vi "T6_E4980A_Correction.vi"(4 "Cable Length (0: 0 m)":u16(ring)=2 items=["0 m"=0, "1 m"=1, "2 m"=2, "4 m"=4], 5 "LCR Correction String":string="CORR:LENG 1;METH MULT;OPEN:STAT ON;:CORR:SHOR:STAT OFF;:CORR:LOAD:STAT OFF;:CORR:SPOT1:STAT ON;FREQ 2E6", 6 "Calib waitTime (ms)":u32=1000, 7 "LCR Setup String":string="FUNC:IMP:TYPE CPQ;RANG:AUTO ON;:FREQ 8E5;VOLT 1;TRIG:SOUR INT;:AMPL:ALC OFF;:APER SHORT,4", 8 "error in":errorcluster, 9 "Relay Definition for Path":string[](array[string])=["C10,C26,C42,C58", "O10,O26,C30,O42,O58,C63", "O10,O26,C30,O42,O58,C63", "O10,O26,C30,O42,O58,C63", "C14,C28,O30,C40,C47,C52,C60,O63", "O14,O28,C31,C40,O47,C52,C54,O60", "C15,C31,C40,C52,C54,C56", "O15,O31,C28,C40,O54,O56,C52,C60", "C28,C40,C52,C60", "C28,C40,C52,C60", "C11,O28,C30,O40,C43,O52,O60,C63", "O11,C26,O30,O43,C58,O63", "C9,O26,C41,O58", "O9,O26,C27,C30,O41,C59,C63", "C13,O27,O30,C40,C46,C52,O59,O63", "C13,C40,C46,C52", "C13,C40,C46,C52", "O13,C29,C31,C40,C52,C54,C61,O46", "C24,C29,C31,C40,C52,C54,C57,C61", "O24,O29,O31,C40,O54,C52,O57,O61", "C12,C27,C30,O40,C44,C59,O52,C63", "C12,C27,C30,O40,C44,C59,O52,C63", "C12,C27,C30,O40,C44,C59,O52,C63", "O9,O26,O10,O36,O11,O27,O12,O40,O14,O31,O13,O28,O15,O29,O24,O41,O58,O42,O60,O63,O43,O59,O44,O52,O46,O60,O47,O54,O56,O61,O57", "C38"], 10 "LCR Meter In":refnum<visa-resource-name>="GPIB0::17::INSTR", 11 "Relay In":refnum<k15>="PXI1Slot2" caption="resource name") -> (0 "error out (no error)":errorcluster, 2 "LCR Out":refnum<visa-resource-name>, 3 "Relay Out":refnum<k15>)   [LabVIEW 2017]
uses:
  <instrlib>/Agilent E4980/Agilent E4980.lvlib
panel:
  in  "T6_Relay Definition for Path":string[](array[string])=["C10,C26,C42,C58", "O10,O26,C30,O42,O58,C63", "C11,O28,C30,O40,C43,O52,O60,C63", "O11,C26,O30,O43,C58,O63", "C38", "O14,O28,C31,C40,O47,C52,C54,O60", "C15,C31,C40,C52,C54,C56", "O15,O31,C28,C40,O54,O56,C52,C60", "C28,C40,C52,C60", "C28,C40,C52,C60", "C11,O28,C30,O40,C43,O52,O60,C63", "O11,C26,O30,O43,C58,O63", "C9,O26,C41,O58", "O9,O26,C27,C30,O41,C59,C63", "C13,O27,O30,C40,C46,C52,O59,O63", "C13,C40,C46,C52", "C13,C40,C46,C52", "O13,C29,C31,C40,C52,C54,C61,O46", "C24,C29,C31,C40,C52,C54,C57,C61", "O24,O29,O31,C40,O54,C52,O57,O61", "C12,C27,C30,O40,C44,C59,O52,C63", "C12,C27,C30,O40,C44,C59,O52,C63", "C12,C27,C30,O40,C44,C59,O52,C63", "O9,O26,O10,O36,O11,O27,O12,O40,O14,O31,O13,O28,O15,O29,O24,O41,O58,O42,O60,O63,O43,O59,O44,O52,O46,O60,O47,O54,O56,O61,O57", "C38"]
  # "Spot 1 --> TMN1.5\nSpot 2 --> VMD"
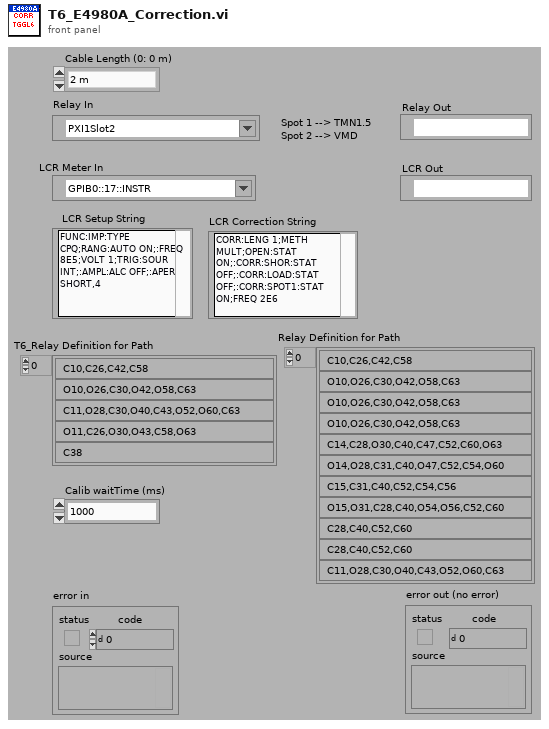
[diagram p1: front panel]
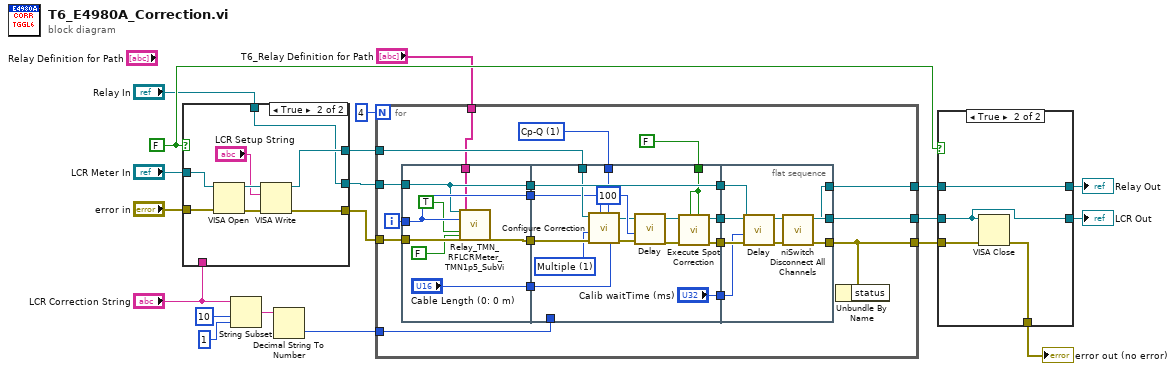
[diagram p0: block diagram]
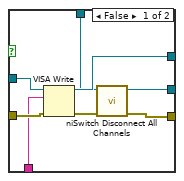
[diagram p3: hidden frame]
diagram:
  w13 = FALSE
  n1 = case shown="True" w13 {
    tunnel: "LCR Meter In" -> [w27 w35]
    tunnel: "error in" -> [w28 w32]
    tunnel: [w26 w31] -> w16
    tunnel: [w22 w29] -> w15
    tunnel: "LCR Correction String" -> [w25 _]
    tunnel: "Relay In" -> [w24 w30]
    tunnel: [w21 w30] -> w6
    frame False {
      n2 = VISA Write(VISA resource name=w27, write buffer=w25, error in (no error)=w28) -> (VISA resource name out=w26:refnum<visa-resource-name>, error out=w23:errorcluster)  [unwired: 1 out]
      n3 = call <instrlib>:"niSwitch Disconnect All Channels.vi"("error in (no error)"=w23, "instrument handle"=w24) -> ("error out"=w22:errorcluster, "instrument handle out"=w21:refnum<k15>)  [unwired: 8 out]
    }
    frame True {
      n4 = VISA Open(error in (no error)=w32, VISA resource name=w35) -> (VISA resource name=w34:refnum<visa-resource-name>, error out=w36:errorcluster)  [unwired: 1 in, 2 out]
      n5 = VISA Write(VISA resource name=w34, write buffer="LCR Setup String", error in (no error)=w36) -> (VISA resource name out=w31:refnum<visa-resource-name>, error out=w29:errorcluster)  [unwired: 1 out]
    }
  }
  n6 = String Subset(string="LCR Correction String", offset (0)=10, length (rest)=1 ("length (rest)")) -> (substring=w9:string)
  n7 = Decimal String To Number(string=w9) -> (number=w8:i32)  [unwired: 3 out]
  n8 = for {
    N: 4 -> [_]
    tunnel: [w37] -> w17
    tunnel: w15 -> [w55]
    tunnel: w16 -> [w52]
    tunnel: [w51] -> w18
    tunnel: w6 -> [w48]
    tunnel: w8 -> [w45]
    tunnel: "T6_Relay Definition for Path" -> [w44]
    tunnel: [w42] -> w4
    i -> [w53]
    w39 = u16 1 items=["Cp-D", "Cp-Q", "Cp-G", "Cp-Rp", "Cs-D", "Cs-Q", "Cs-Rs", "Lp-D", "Lp-Q", "Lp-G", "Lp-Rp", "Ls-D", "Ls-Q", "Ls-Rs", "R-X", "Z-thd", "Z-thr", "G-B", "Y-thd", "Y-thr"] ("Load Type (0: Cp-D)")
    n9 = flat-sequence {
      tunnel: w53 -> [w61]
      tunnel: w48 -> [w58]
      tunnel: w55 -> [w63]
      tunnel: [w62] -> w54
      tunnel: [w61] -> w50
      tunnel: [w58] -> w46
      tunnel: w44 -> [w57]
      tunnel: ["Cable Length (0: 0 m)"] -> w38
      tunnel: w54 -> [w75]
      tunnel: w52 -> [w69]
      tunnel: w50 -> [w67]
      tunnel: [w72] -> w49
      tunnel: FALSE ("Short Corr (T: On)") -> [w64]
      tunnel: [w78] -> w47
      tunnel: w46 -> [w78]
      tunnel: w45 -> [_]
      tunnel: ["Calib waitTime (ms)"] -> w41
      tunnel: [w71] -> w40
      tunnel: w39 -> [w68]
      tunnel: w38 -> [w65]
      tunnel: [w85] -> w51
      tunnel: [w82] -> w37
      tunnel: [w81] -> w42
      tunnel: w40 -> [w85]
      tunnel: w41 -> [w79]
      tunnel: w47 -> [w84]
      tunnel: w49 -> [w80]
      frame #0 {
        n10 = call "Relay_TMN_RFLCRMeter_TMN1p5_SubVi.vi"("resource name"=w58, "Device List"=w61, "PUSH BUTTON TO EXECUTE"=TRUE, "CLICK DOWN TO QUIT"=FALSE ("PUSH BUTTON TO EXECUTE"), "errorin"=w63, "Relay Definition for Path"=w57) -> ("error out"=w62:errorcluster)  [unwired: 7 in, 14 out]
      }
      frame #1 {
        w66 = u16 1 items=["Single", "Multiple"] ("Correction Mode (0: Single)")
        n11 = call <instrlib>:"Configure Correction.vi"("Load Type (0: Cp-D)"=w68, "Channel Number (0)"=w67, "error in (no error)"=w75, "Correction Mode (0: Single)"=w66, "Cable Length (0: 0 m)"=w65, "VISA resource name"=w69) -> ("error out"=w74:errorcluster, "VISA resource name out"=w70:refnum<visa-resource-name>)  [unwired: 4 in]
        n12 = call "Delay.vi"("error in (no error)"=w74, "Delay"=u32 100) -> ("error out"=w73:errorcluster)  [unwired: 9 in]
        n13 = call <instrlib>:"Execute Spot Correction.vi"("Load Correction (T:Yes)"=w64, "Short Correction (T:Yes)"=w64, "error in (no error)"=w73, "VISA resource name"=w70) -> ("error out"=w72:errorcluster, "VISA resource name out"=w71:refnum<visa-resource-name>)  [unwired: 6 in]
      }
      frame #2 {
        n14 = call "Delay.vi"("error in (no error)"=w80, "Delay"=w79) -> ("error out"=w83:errorcluster)  [unwired: 9 in]
        n15 = call <instrlib>:"niSwitch Disconnect All Channels.vi"("error in (no error)"=w83, "instrument handle"=w84) -> ("error out"=w82:errorcluster, "instrument handle out"=w81:refnum<k15>)  [unwired: 8 out]
      }
    }
    n16 = Unbundle By Name(w37) -> ()  [unwired: 1 out]
  }
  n17 = case shown="True" w13 {
    tunnel: w18 -> [w86 w89]
    tunnel: w17 -> [w88 w92]
    tunnel: [w88 w91] -> w14
    tunnel: w4 -> [w87 w90]
    tunnel: [w87 w90] -> w3
    tunnel: [w86 w89] -> w2
    frame False {
    }
    frame True {
      n18 = VISA Close(VISA resource name=w89, error in (no error)=w92) -> (error out=w91:errorcluster)
    }
  }
  "error out (no error)" <- w14
  "Relay Out" <- w3
  "LCR Out" <- w2
